vi "SGUI Example - string assign.vi"() -> ()   [LabVIEW 2020, in "varilib.lvlib"]
uses:
  varilib.lvlib
  SGUI Assign Single String With Tags.vi
  SGUI Assign Multiple Strings With Tags.vi
panel:
  out "str line 3":string
  out "str line 2":string
  out "str line 1":string
  out "Formatted String (all rows of text to one control)":string
  in  "input string":string="This is a plain string line.\n<b>This is a <tc=0000FF>bold</tc> string line.</b>\n<i>This is an italic string line.</i>\nVlozenej radek voe\n<u>This is an underline</u> string line\n<s>This is a <tc=red>strikeout</tc> string line.</s>\n\n<b><i><u><s>This is an all above formatted string line.</s></u></i></b>\n\nThis is a plain string line."
  # "text split per\nrows to separate\ncontrols"
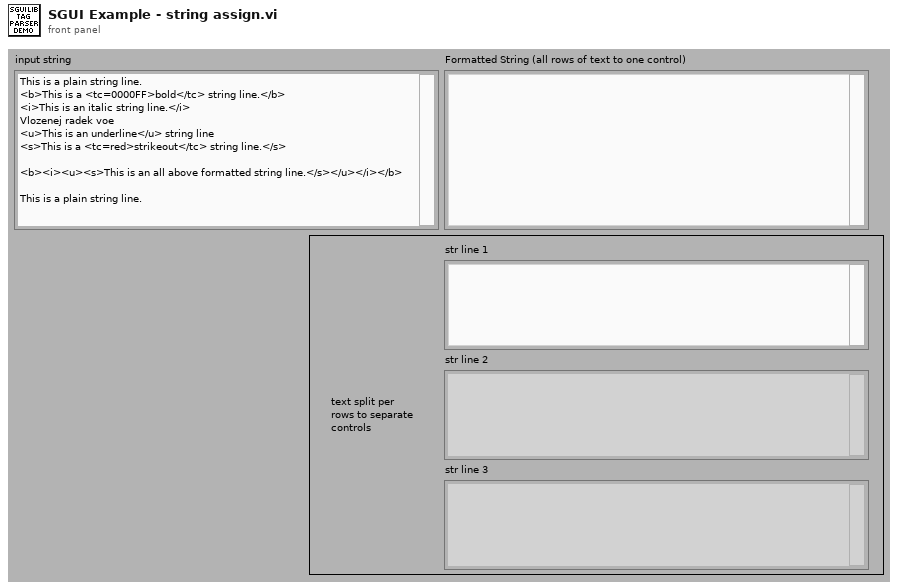
[diagram p1: front panel]
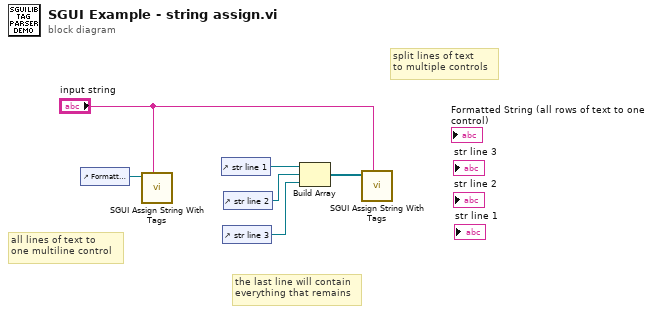
[diagram p0: block diagram]
diagram:
  # "the last line will contain\neverything that remains"
  # "split lines of text\nto multiple controls"
  # "all lines of text to\none multiline control"
  n1 = control-ref of="Formatted String (all rows of text to one control)"() -> (w3:refnum<vi>)
  n2 = call-poly "SGUI Assign String With Tags.vi"("string ref"=w3, "string (empty)"="input string") -> ()  [unwired: 8 in, 2 out]
  n3 = control-ref of="str line 1"() -> (w6:refnum<vi>)
  n4 = control-ref of="str line 3"() -> (w4:refnum<vi>)
  n5 = control-ref of="str line 2"() -> (w5:refnum<vi>)
  n6 = Build Array(w6, w5, w4) -> (w2:refnum<vi>[])
  n7 = call-poly "SGUI Assign String With Tags.vi"("string refs"=w2, "string (empty)"="input string") -> ()  [unwired: 8 in, 2 out]
